vi "PCA9685 Servo Test.vi"() -> ()   [LabVIEW 2020]
uses:
  <vilib>/MakerHub/LINX/LMH-LINX.lvlib
  LINX-PCA9685 PWM/LINX-PCA9685 PWM.lvclass
  LINX I2C/LINX I2C.lvclass
  <vilib>/MakerHub/LINX/Public/Utilities/Open Local.vi
panel:
  in  "PWM1":dbl(slide) scale=-100.0..100.0
  in  "PWM0":dbl(slide) scale=-100.0..100.0
  out "New Frequency (Hz)":dbl
  out "Initial Frequency (Hz)":dbl
  in  "stop":bool
  out "Error Out":errorcluster
  # "A simple example of driving two servo motors with a Raspberry Pi using the PCA9685 PWM driver chip.\n\nThe board provides 16 PWM channels for driving LEDs or Servos."
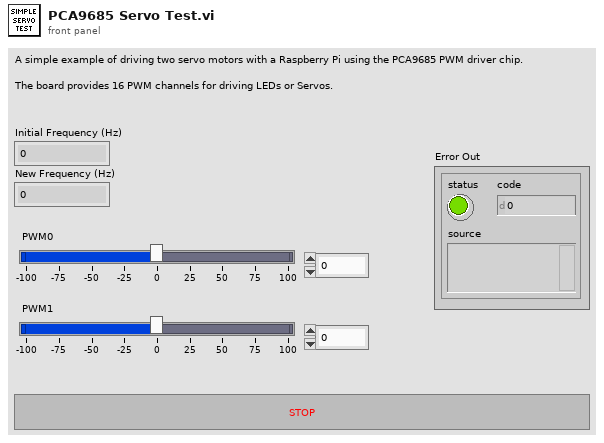
[diagram p1: front panel]
types:
  T1 = typedef "LMH-LINX.lvlib/LINX Ref.ctl" = cluster{"IO":T2, "Interface":T3, "LINX Device Config":T4}
  T2 = typedef "LMH-LINX.lvlib/Platform.ctl" = enum16{"Remote", "Local"}
  T3 = typedef "LMH-LINX.lvlib/Interface.ctl" = enum16{"Serial", "TCP"}
  T4 = typedef "LMH-LINX.lvlib/Device.lvlib/LINX Device Config.ctl" = cluster{"Interface":T3, "COM Port":refnum<visa-resource-name>, "TCP Configuration":T5, "Device Family":u8, "Device ID":u8, "Device Name":string, "TCP Ref":refnum<k5>, "Channels":T6}
  T5 = typedef "LMH-LINX.lvlib/Device.lvlib/TCP Config.ctl" = cluster{"IP Address":string, "Port":u16}
  T6 = typedef "LMH-LINX.lvlib/Channels.ctl" = cluster{"DI":u8[], "DO":u8[], "AI":u8[], "AO":u8[], "PWM":u8[], "QE":u8[], "UART":u8[], "I2C 2":u8[], "SPI":u8[], "CAN":u8[], "Servo":u8[], "AI Ref (V)":dbl, "AI Resolution (Bits)":u8, "AO Ref (V)":dbl, "AO Resolution (Bits)":u8}
  T7 = enum16{"LED/PWM00", "LED/PWM01", "LED/PWM02", "LED/PWM03", "LED/PWM04", "LED/PWM05", "LED/PWM06", "LED/PWM07", "LED/PWM08", "LED/PWM09", "LED/PWM10", "LED/PWM11", "LED/PWM12", "LED/PWM13", "LED/PWM14", "LED/PWM15"}[]
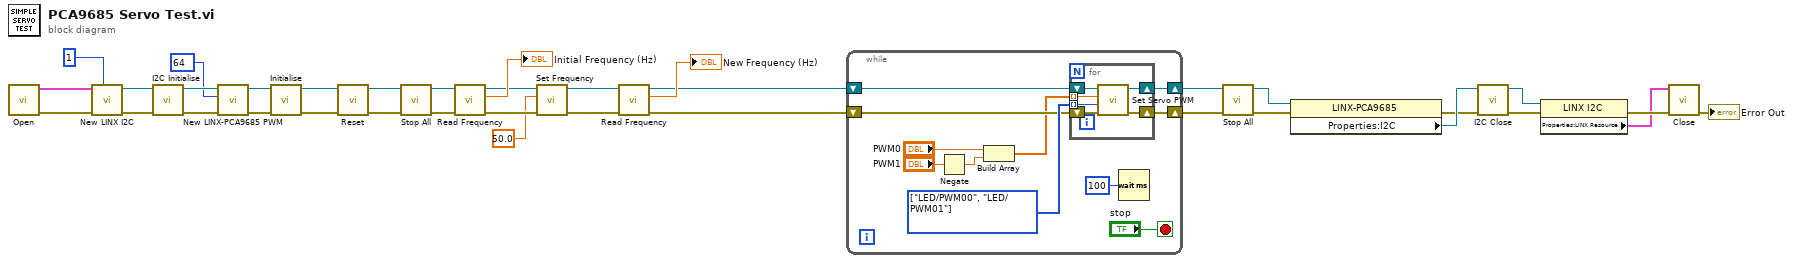
[diagram p0: block diagram]
diagram:
  n1 = call-poly <vilib>:"Open.vi"() -> ("Error Out"=w15:errorcluster, "LINX Resource"=w16:T1)  [unwired: 9 in, 1 out]
  n2 = call "New LINX I2C.vi"("LINX I2C Channel"=u8 1 ("I2C Channel"), "error in (no error)"=w15, "LINX Resource"=w16) -> ("error out"=w13:errorcluster, "LINX I2C out"=w12:refnum<class "LINX I2C.lvclass">)  [unwired: 7 in]
  n3 = call-dynamic "I2C Initialise.vi"("error in (no error)"=w13, "LINX I2C in"=w12) -> ("error out"=w5:errorcluster, "LINX I2C out"=w4:refnum<class "LINX I2C.lvclass">)  [unwired: 8 in]
  n4 = call "New LINX-PCA9685 PWM.vi"("error in (no error)"=w5, "I2C Slave Address (0x40)"=u8 64, "I2C"=w4) -> ("error out"=w3:errorcluster, "LINX-PCA9865 PWM out"=w2:refnum<class "LINX-PCA9685 PWM.lvclass">)  [unwired: 7 in]
  n5 = call-dynamic "Initialise.vi"("error in (no error)"=w3, "PWM in"=w2) -> ("error out"=w20:errorcluster, "PWM out"=w21:refnum<class "LINX-PCA9685 PWM.lvclass">)  [unwired: 8 in]
  n6 = call-dynamic "Reset.vi"("error in (no error)"=w20, "PWM in"=w21) -> ("error out"=w19:errorcluster, "PWM out"=w18:refnum<class "LINX-PCA9685 PWM.lvclass">)  [unwired: 8 in]
  n7 = call-dynamic "Stop All.vi"("error in (no error)"=w19, "LINX-PCA9865 PWM in"=w18) -> ("error out"=w28:errorcluster, "LINX-PCA9865 PWM out"=w29:refnum<class "LINX-PCA9685 PWM.lvclass">)  [unwired: 8 in]
  n8 = call-dynamic "Read Frequency.vi"("error in (no error)"=w28, "PWM in"=w29) -> ("error out"=w34:errorcluster, "Frequency (Hz)"=→"Initial Frequency (Hz)":dbl, "PWM out"=w33:refnum<class "LINX-PCA9685 PWM.lvclass">)  [unwired: 7 in]
  n9 = call-dynamic "Set Frequency.vi"("error in (no error)"=w34, "Frequency (1000Hz)"=50.0, "PWM in"=w33) -> ("error out"=w32:errorcluster, "PWM out"=w31:refnum<class "LINX-PCA9685 PWM.lvclass">)  [unwired: 7 in]
  n10 = call-dynamic "Read Frequency.vi"("error in (no error)"=w32, "PWM in"=w31) -> ("error out"=w25:errorcluster, "Frequency (Hz)"=→"New Frequency (Hz)":dbl, "PWM out"=w26:refnum<class "LINX-PCA9685 PWM.lvclass">)  [unwired: 7 in]
  n11 = while {
    shift-right: [w44] -> w27
    shift-left: w25 -> [w41]
    shift-right: [w43] -> w24
    shift-left: w26 -> [w45]
    stop <- "stop" stop-if-true
    w42 = T7 [enum."LED/PWM00", enum."LED/PWM01"] items=["LED/PWM00", "LED/PWM01", "LED/PWM02", "LED/PWM03", "LED/PWM04", "LED/PWM05", "LED/PWM06", "LED/PWM07", "LED/PWM08", "LED/PWM09", "LED/PWM10", "LED/PWM11", "LED/PWM12", "LED/PWM13", "LED/PWM14", "LED/PWM15"] ("LEDn (PWM channel)")
    n12 = Negate(x="PWM1") -> (-x=w38:dbl)
    n13 = Build Array("PWM0", w38) -> (w37:dbl[])
    n14 = for {
      tunnel: w37 -> [w50] mode=indexing
      tunnel: w42 -> [w49] mode=indexing
      shift-right: [w51] -> w43
      shift-left: w45 -> [w53]
      shift-right: [w52] -> w44
      shift-left: w41 -> [w48]
      n15 = call "Set Servo PWM.vi"("error in (no error)"=w48, "LEDn (PWM channel)"=w49, "Servo Speed (-100 to 100%)"=w50, "LINX-PCA9865 PWM in"=w53) -> ("error out"=w52:errorcluster, "LINX-PCA9865 PWM out"=w51:refnum<class "LINX-PCA9685 PWM.lvclass">)  [unwired: 6 in]
    }
    n16 = Wait (ms)(milliseconds to wait=u32 100) -> ()  [unwired: 1 out]
  }
  n17 = call-dynamic "Stop All.vi"("error in (no error)"=w27, "LINX-PCA9865 PWM in"=w24) -> ("error out"=w22:errorcluster, "LINX-PCA9865 PWM out"=w23:refnum<class "LINX-PCA9685 PWM.lvclass">)  [unwired: 8 in]
  n18 = property class="LINX-PCA9685"(reference=w23, error in=w22) -> (error out=w10:errorcluster, "Properties:I2C"=w11:refnum<class "LINX I2C.lvclass">)  [unwired: 1 out]
  n19 = call-dynamic "I2C Close.vi"("error in (no error)"=w10, "LINX I2C in"=w11) -> ("error out"=w9:errorcluster, "LINX I2C out"=w7:refnum<class "LINX I2C.lvclass">)  [unwired: 8 in]
  n20 = property class="LINX I2C"(reference=w7, error in=w9) -> (error out=w8:errorcluster, "Properties:LINX Resource"=w6:T1)  [unwired: 1 out]
  n21 = call <vilib>:"Close.vi"("Error In"=w8, "LINX Resource"=w6) -> ("Error Out"=→"Error Out":errorcluster)  [unwired: 9 in]
